vi "Alarme temperatura.vi"() -> ()   [LabVIEW 2018]
panel:
  in  "Alarme aos:":dbl
  in  "Escala":bool
  out "TEMP Historical":cluster{dbl, "Thermometer":dbl, "Limite":dbl}(graph)
  in  "POWER":bool
  # "ON"
  # "OFF"
  # "Celsius"
  # "Fahreneit"
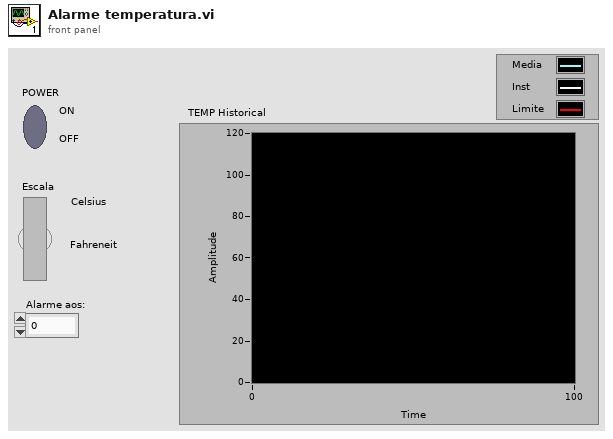
[diagram p1: front panel]
types:
  T1 = cluster{dbl, "Thermometer":dbl, "Alarme aos:":dbl}
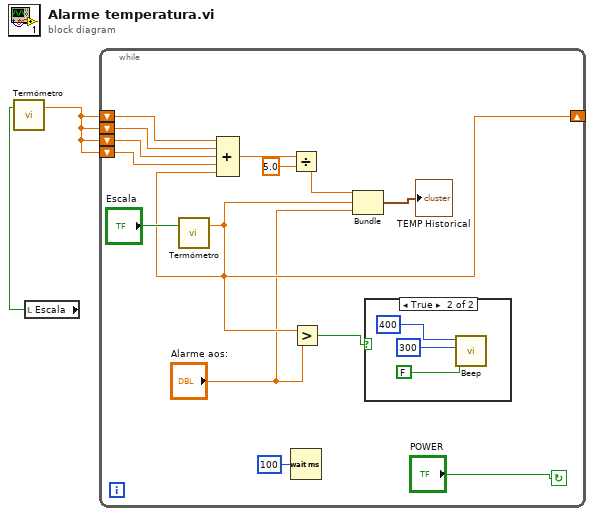
[diagram p0: block diagram]
diagram:
  n1 = local read "Escala"() -> (w1:bool)
  n2 = call "Termómetro.vi"("Temp Scale"=w1) -> ("Thermometer"=w2:dbl)  [unwired: 2 in]
  n3 = while {
    shift-right: [w5] -> _
    shift-left: w2 -> [w13]
    shift-left: w2 -> [w12]
    shift-left: w2 -> [w10]
    shift-left: w2 -> [w11]
    stop <- "POWER" continue-if-true
    n4 = call "Termómetro.vi"("Temp Scale"="Escala") -> ("Thermometer"=w5:dbl)  [unwired: 2 in]
    n5 = Compound Arithmetic op=ADD(w13, w12, w11, w10, w5) -> (w9:dbl)
    n6 = Divide(x=w9, y=5.0) -> (x/y=w7:dbl)
    n7 = Wait (ms)(milliseconds to wait=u32 100) -> ()  [unwired: 1 out]
    n8 = Greater?(x=w5, y="Alarme aos:") -> (0:w4:bool)
    n9 = Bundle(w7, "Thermometer"=w5, "Alarme aos:"="Alarme aos:") -> (→"TEMP Historical":T1)  [unwired: 1 in]
    n10 = case shown="True" w4 {
      frame False {
      }
      frame True {
        n11 = call <vilib>:"Beep.vi"("use system alert? (T)"=FALSE, "duration (msec)"=u32 300, "frequency (Hz)"=u32 400) -> ()  [unwired: 9 in]
      }
    }
  }
